vi "Car Wash Controller.vi"(8 "error in (no error)":errorcluster, 11 "View Model":T1) -> (0 "error out":errorcluster, 3 "View Model":T1)   [LabVIEW 2017]
doc: "This SW component allows the user to interact with the controls and provides appropriate feedback as requested through the display console."
uses:
  View Model/Controls/View Model.ctl
  View Model/Controls/Shared Model.ctl
  Error Handler/Controls/Error Model.ctl
  Error Handler/Controls/Error Data.ctl
  Error Handler/Controls/Error Level.ctl
  Configuration/Controls/Config Model.ctl
  Configuration/Controls/Config Record.ctl
  Configuration/Controls/Config Data.ctl
  Configuration/Controls/Config Command.ctl
  Controls/Controler Model.ctl
  Views/Entry Console View/Controls/Entry Console - Wash Steps.ctl
  Controls/Controller - Event.ctl
  Controls/Controller - Commands.ctl
  Controls/Controller - Overhead.ctl
  Controls/Controller - States.ctl
  Controls/Controller - Wash Step.ctl
  Views/Vehicle Position View/Controls/Vehicle - Station Enum.ctl
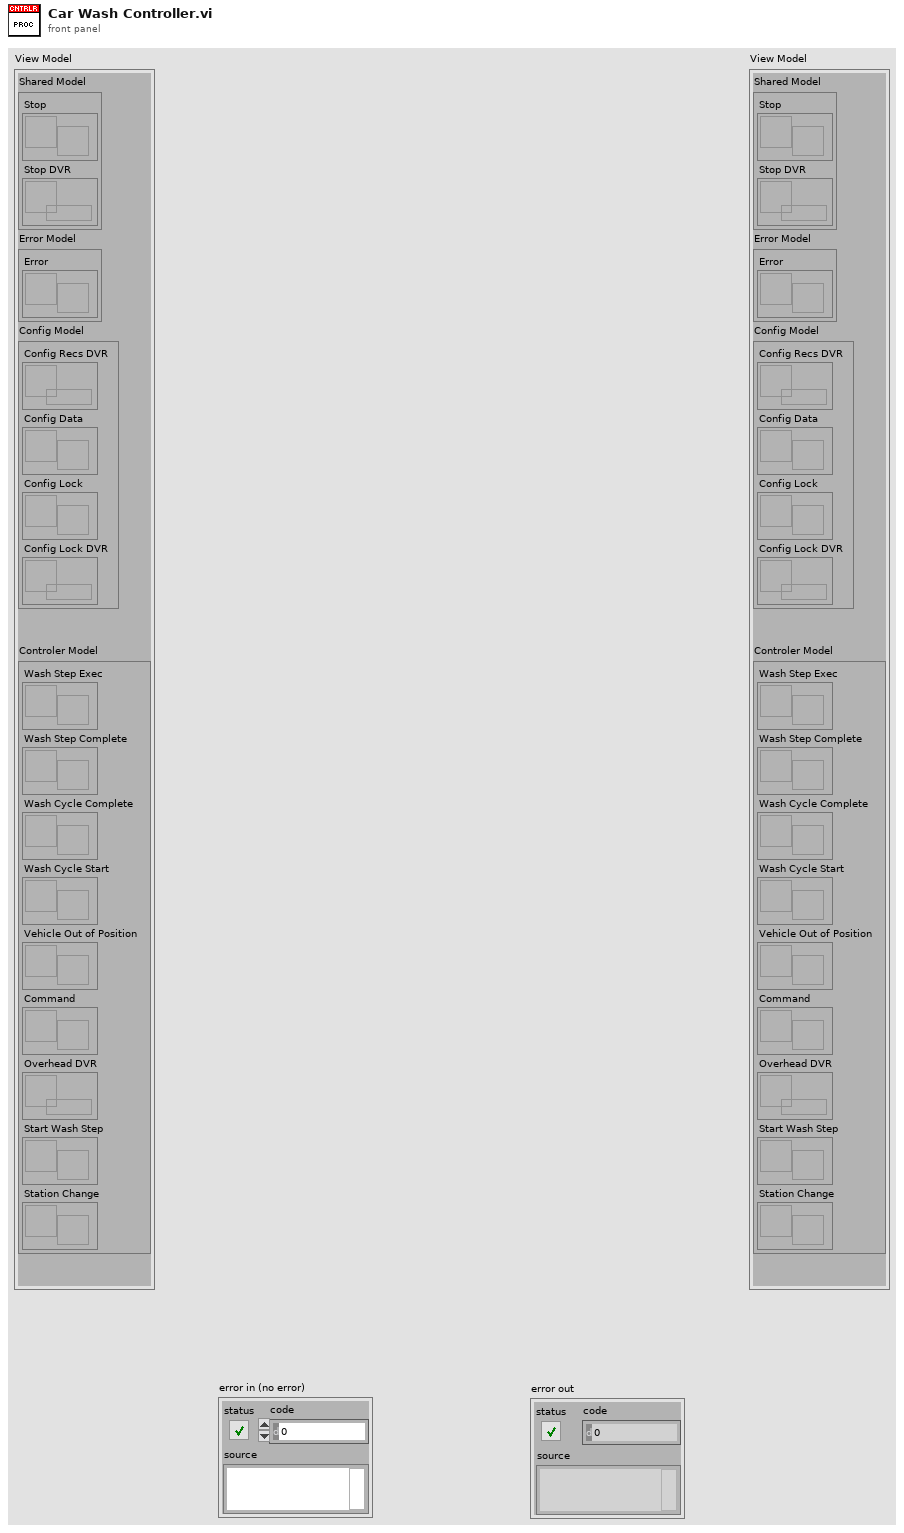
[diagram p1: front panel]
types:
  T1 = typedef "View Model.ctl" = cluster{"Shared Model":T2, "Error Model":T3, "Config Model":T4, "Controler Model":T5}
  T2 = typedef "Shared Model.ctl" = cluster{"Stop":refnum<user-event>, "Stop DVR":refnum<data-value>}
  T3 = typedef "Error Model.ctl" = cluster{"Error":refnum<user-event>}
  T4 = typedef "Config Model.ctl" = cluster{"Config Recs DVR":refnum<data-value>, "Config Data":refnum<user-event>, "Config Lock":refnum<user-event>, "Config Lock DVR":refnum<data-value>}
  T5 = typedef "Controler Model.ctl" = cluster{"Wash Step Exec":refnum<user-event>, "Wash Step Complete":refnum<user-event>, "Wash Cycle Complete":refnum<user-event>, "Wash Cycle Start":refnum<user-event>, "Vehicle Out of Position":refnum<user-event>, "Command":refnum<user-event>, "Overhead DVR":refnum<data-value>, "Start Wash Step":refnum<user-event>, "Station Change":refnum<user-event>}
  T6 = typedef "Config Command.ctl" = enum16{"Read", "Query", "Insert", "Update"}
  T7 = typedef "Controller - States.ctl" = enum16{"Initial", "Wait for Start", "Wash Cycle Start", "Wait for Vehicle Position", "Wash Step Start", "Wash Step Execute", "Wash Step Complete", "Wash Cycle Complete", "Wash Exit", "Wash Abort/Terminate"}
  T8 = typedef "Error Level.ctl" = enum16{"Minor Error", "Wash Cycle Error", "System Error"}
  T9 = typedef "Controller - Commands.ctl" = enum16{"Start Wash Cycle", "Finish Wash Cycle", "Start Wash Step", "Execute Wash Step", "Finish Wash Step", "Wash Terminate"}
  T10 = typedef "Controller - Wash Step.ctl" = enum16{"Under Body Wash", "Bug Remover", "Pre-Soak", "High Pressure Wash", "Low Pressure Wax", "Spot Free Rinse", "Tire Shine Foam", "Air Dry"}
  T11 = typedef "Vehicle - Station Enum.ctl" = enum16{"Entry", "Station1", "Station2", "Station3", "Exit"}
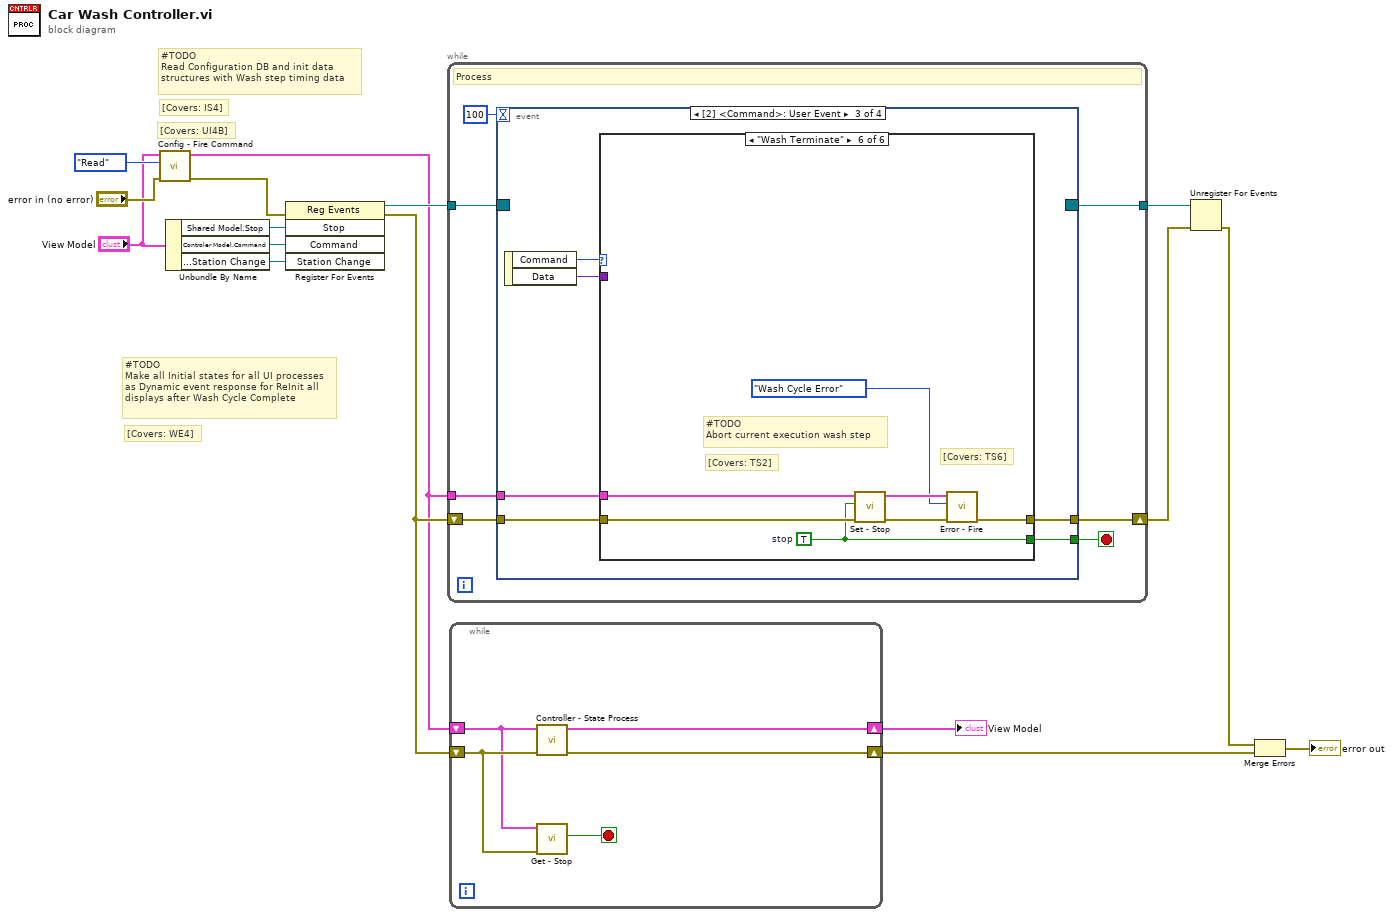
[diagram p0: block diagram]
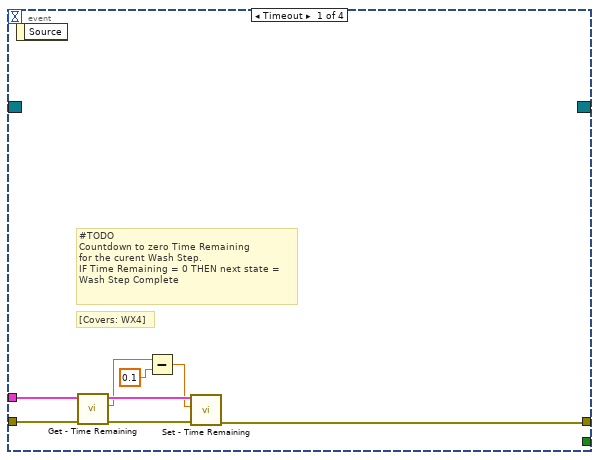
[diagram p2: hidden frame]
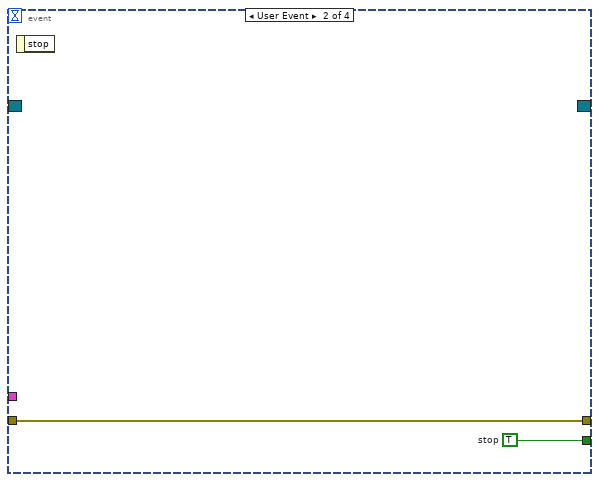
[diagram p3: hidden frame]
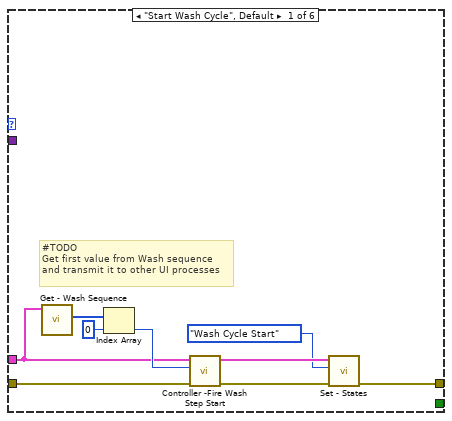
[diagram p4: hidden frame]
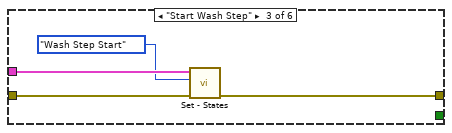
[diagram p6: hidden frame]
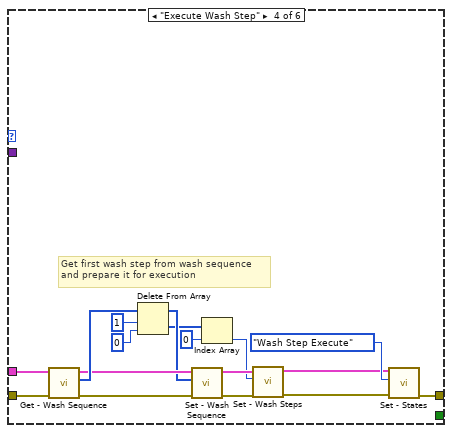
[diagram p7: hidden frame]
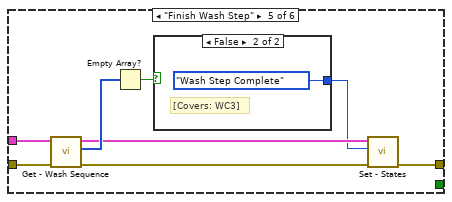
[diagram p8: hidden frame]
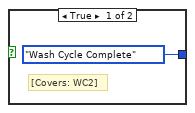
[diagram p9: hidden frame]
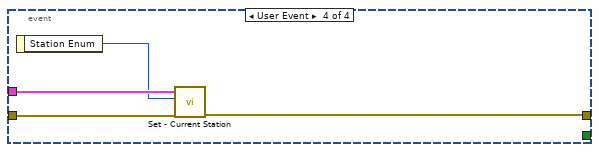
[diagram p10: hidden frame]
diagram:
  # "[Covers: WE4]"
  # "#TODO\nMake all Initial states for all UI processes\nas Dynamic event response for ReInit all\ndisplays after Wash Cycle Complete"
  # "[Covers: UI4B]"
  # "[Covers: IS4]"
  # "#TODO\nRead Configuration DB and init data\nstructures with Wash step timing data"
  n1 = call "Config - Fire Command.vi"("error in (no error)"="error in (no error)", "Config Command"=Config_Command."Read", "View Model"="View Model") -> ("error out"=w2:errorcluster, "View Model"=w1:T1)  [unwired: 7 in]
  n2 = Unbundle By Name("View Model") -> ("Shared Model.Stop"=w16:refnum<user-event>, "Controler Model.Command"=w7:refnum<user-event>, "Controler Model.Station Change"=w6:refnum<user-event>)
  n3 = register-events(error in=w2, w16, w7, w6) -> (reference out=w15:refnum<event-registration>, error out=w12:errorcluster)  [unwired: 1 in]
  n4 = while {
    tunnel: w15 -> [w23]
    shift-right: [w21] -> w13
    shift-left: w12 -> [w22]
    tunnel: [w19] -> w14
    tunnel: w1 -> [w18]
    stop <- w20 stop-if-true
    # "Process"
    n5 = event shown="[2] <Command>: User Event" {
      selector: w23 -> [_ _ _ _]
      dyn-events: [_ _ _ _] -> w19
      timeout: 100 -> [_ _ _ _]
      tunnel: w22 -> [w31 w33 w37 w91]
      tunnel: [w28 w33 w35 w88] -> w21
      tunnel: [_ w32 w34 _] -> w20
      tunnel: w18 -> [w30 _ w36 w90]
      event Timeout {
        # "[Covers: WX4]"
        # "#TODO\nCountdown to zero Time Remaining\nfor the curent Wash Step.\nIF Time Remaining = 0 THEN next state =\nWash Step Complete"
        n6 = event-data() -> ()  [unwired: 1 in, 1 out]
        n7 = call "Get - Time Remaining.vi"("error in (no error)"=w31, "View Model"=w30) -> ("error out"=w29:errorcluster, "Elapsed Time"=w26:dbl, "View Model"=w27:T1)  [unwired: 7 in]
        n8 = Subtract(x=w26, y=0.1) -> (x-y=w24:dbl)
        n9 = call "Set - Time Remaining.vi"("error in (no error)"=w29, "Elapsed Time"=w24, "View Model"=w27) -> ("error out"=w28:errorcluster)  [unwired: 7 in, 1 out]
      }
      event User Event {
        w32 = TRUE  # stop
        n10 = event-data() -> ()  [unwired: 1 in, 1 out]
      }
      event User Event {
        n11 = event-data() -> ("Command"=w39:T9, "Data"=w38:variant)  [unwired: 1 in]
        n12 = case shown="\"Wash Terminate\"" w39 {
          tunnel: w38 -> [_ _ _ _ _ _]
          tunnel: w37 -> [w45 w49 w53 w68 w78 w87]
          tunnel: w36 -> [w44 _ w51 w67 w77 w86]
          tunnel: [w41 w49 w52 w70 w73 w83] -> w35
          tunnel: [_ _ _ _ _ w85] -> w34
          frame "Start Wash Cycle", Default {
            # "#TODO\nGet first value from Wash sequence\nand transmit it to other UI processes"
            n13 = call "Get - Wash Sequence.vi"("View Model"=w44) -> ("Wash Sequence"=w47:T10[])  [unwired: 8 in, 2 out]
            n14 = Index Array(array=w47, index=0) -> (element=w46:T10)
            n15 = call "Controller -Fire Wash Step Start.vi"("error in (no error)"=w45, "Wash Step"=w46, "View Model"=w44) -> ("error out"=w43:errorcluster, "View Model"=w42:T1)  [unwired: 7 in]
            n16 = call "Set - States.vi"("error in (no error)"=w43, "Current State"=Controller_-_States."Wash Cycle Start", "View Model"=w42) -> ("error out"=w41:errorcluster)  [unwired: 7 in, 1 out]
          }
          frame "Finish Wash Cycle" {
          }
          frame "Start Wash Step" {
            n17 = call "Set - States.vi"("error in (no error)"=w53, "Current State"=Controller_-_States."Wash Step Start", "View Model"=w51) -> ("error out"=w52:errorcluster)  [unwired: 7 in, 1 out]
          }
          frame "Execute Wash Step" {
            # "Get first wash step from wash sequence\nand prepare it for execution"
            n18 = call "Get - Wash Sequence.vi"("error in (no error)"=w68, "View Model"=w67) -> ("error out"=w62:errorcluster, "Wash Sequence"=w66:T10[], "View Model"=w63:T1)  [unwired: 7 in]
            n19 = Delete From Array(array=w66, length=1, index=0) -> (deleted portion=w58:T10[], array with subset deleted=w61:T10[])
            n20 = call "Set - Wash Sequence.vi"("error in (no error)"=w62, "Wash Sequence"=w61, "View Model"=w63) -> ("error out"=w60:errorcluster, "View Model"=w59:T1)  [unwired: 7 in]
            n21 = Index Array(array=w58, index=0) -> (element=w56:T10)
            n22 = call "Set - Wash Steps.vi"("error in (no error)"=w60, "Current Wash Step"=w56, "View Model"=w59) -> ("error out"=w55:errorcluster, "View Model"=w54:T1)  [unwired: 7 in]
            n23 = call "Set - States.vi"("error in (no error)"=w55, "Current State"=Controller_-_States."Wash Step Execute", "View Model"=w54) -> ("error out"=w70:errorcluster)  [unwired: 7 in, 1 out]
          }
          frame "Finish Wash Step" {
            n24 = call "Get - Wash Sequence.vi"("error in (no error)"=w78, "View Model"=w77) -> ("error out"=w74:errorcluster, "Wash Sequence"=w76:T10[], "View Model"=w72:T1)  [unwired: 7 in]
            n25 = Empty Array?(array=w76) -> (empty?=w75:bool)
            n26 = case shown="False" w75 {
              tunnel: [Controller_-_States."Wash Cycle Complete" ("Current State") Controller_-_States."Wash Step Complete" ("Current State")] -> w71
              frame True {
                # "[Covers: WC2]"
              }
              frame False {
                # "[Covers: WC3]"
              }
            }
            n27 = call "Set - States.vi"("error in (no error)"=w74, "Current State"=w71, "View Model"=w72) -> ("error out"=w73:errorcluster)  [unwired: 7 in, 1 out]
          }
          frame "Wash Terminate" {
            w85 = TRUE  # stop
            # "[Covers: TS6]"
            # "[Covers: TS2]"
            # "#TODO\nAbort current execution wash step"
            n28 = call "Set - Stop.vi"("error in (no error)"=w87, "Stop"=w85, "View Model"=w86) -> ("error out"=w84:errorcluster, "View Model"=w82:T1)  [unwired: 7 in]
            n29 = call "Error - Fire.vi"("error in (no error)"=w84, "Error Level"=Error_Level."Wash Cycle Error", "View Model"=w82) -> ("error out"=w83:errorcluster)  [unwired: 7 in, 1 out]
          }
        }
      }
      event User Event {
        n30 = event-data() -> ("Station Enum"=w89:T11)  [unwired: 1 in]
        n31 = call "Set - Current Station.vi"("error in (no error)"=w91, "Current Station"=w89, "View Model"=w90) -> ("error out"=w88:errorcluster)  [unwired: 7 in, 1 out]
      }
    }
  }
  n32 = while {
    shift-right: [w92] -> w8
    shift-left: w1 -> [w94]
    shift-right: [w93] -> w11
    shift-left: w12 -> [w95]
    stop <- w96 stop-if-true
    n33 = call "Controller - State Process.vi"("error in (no error)"=w95, "View Model"=w94) -> ("error out"=w93:errorcluster, "View Model"=w92:T1)  [unwired: 8 in]
    n34 = call "Get - Stop.vi"("error in (no error)"=w95, "View Model"=w94) -> ("Stop"=w96:bool)  [unwired: 7 in, 2 out]
  }
  "View Model" <- w8
  n35 = Unregister For Events(event registration refnum=w14, error in=w13) -> (error out=w10:errorcluster)
  n36 = Merge Errors(w10, w11) -> (→"error out":errorcluster)
